vi "XY Graph Get Plot Names & Number.vi"(8 "error in (no error)":errorcluster, 11 "XYGraph in":T1) -> (0 "error out":errorcluster, 1 "# Plots":i32, 2 "Plot Names":string[](array[string]), 3 "XYGraph out":T1, 4 "Empty Plots?":bool[](array[boolean]))   [LabVIEW 2019]
uses:
  XY Graph Refnum.ctl
  XY Graph Add-Ons.lvlib
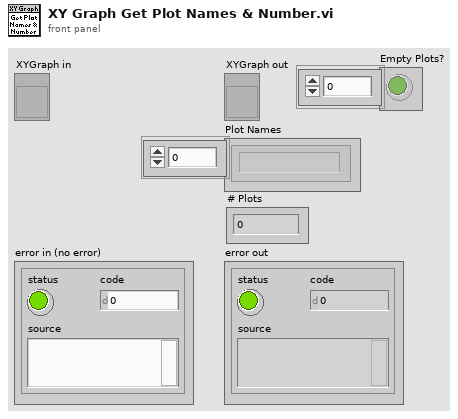
[diagram p1: front panel]
types:
  T1 = typedef "XY Graph Add-Ons.lvlib/XY Graph Refnum.ctl" = refnum<vi>
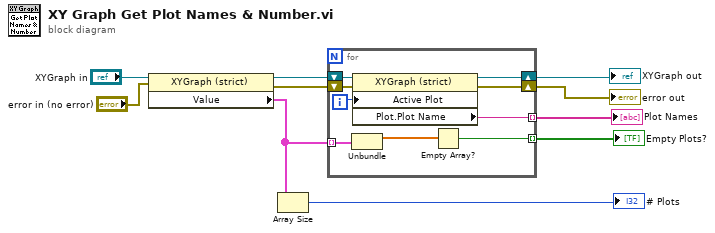
[diagram p0: block diagram]
diagram:
  n1 = property class="XYGraph (strict)"(reference="XYGraph in", error in="error in (no error)") -> (reference out=w7:T1, error out=w5:errorcluster, "Value"=w2:cluster{"X Array":dbl[], "Y Array":dbl[]}[])
  n2 = Array Size(array=w2) -> (size(s)=→"# Plots":i32)
  n3 = for {
    shift-right: [w18] -> w9
    shift-left: w7 -> [w19]
    shift-right: [w14] -> w10
    shift-left: w5 -> [w17]
    tunnel: [w15] -> w3 mode=indexing
    tunnel: w2 -> [w13] mode=indexing
    tunnel: [w11] -> w1 mode=indexing
    i -> [w16]
    n4 = Unbundle(w13) -> ("X Array"=w12:dbl[])  [unwired: 1 out]
    n5 = property class="XYGraph (strict)"(reference=w19, error in=w17, "Active Plot"=w16) -> (reference out=w18:T1, error out=w14:errorcluster, "Plot.Plot Name"=w15:string)
    n6 = Empty Array?(array=w12) -> (empty?=w11:bool)
  }
  "error out" <- w10
  "XYGraph out" <- w9
  "Plot Names" <- w3
  "Empty Plots?" <- w1
